vi "NumberOfPhases.vi"(11 "Device(s)Settings":T1 {"Phase Select" items=["Phase ALL", "Phase A", "Phase B", "Phase C"]}) -> (2 "Numeric Indicator":i32, 3 "Error Out":errorcluster, 5 "Boolean":bool)   [LabVIEW 2018, in "AcPwrPlugins.lvlib" / "NHRDCPower.lvclass"]
uses:
  NHRDCPower.lvclass
  TypeDefs/Device(s)Settings.ctl
  <vilib>/Utility/error.llb/Error Cluster From Error Code.vi
  <vilib>/ErrorRing/Error Ring.xnode
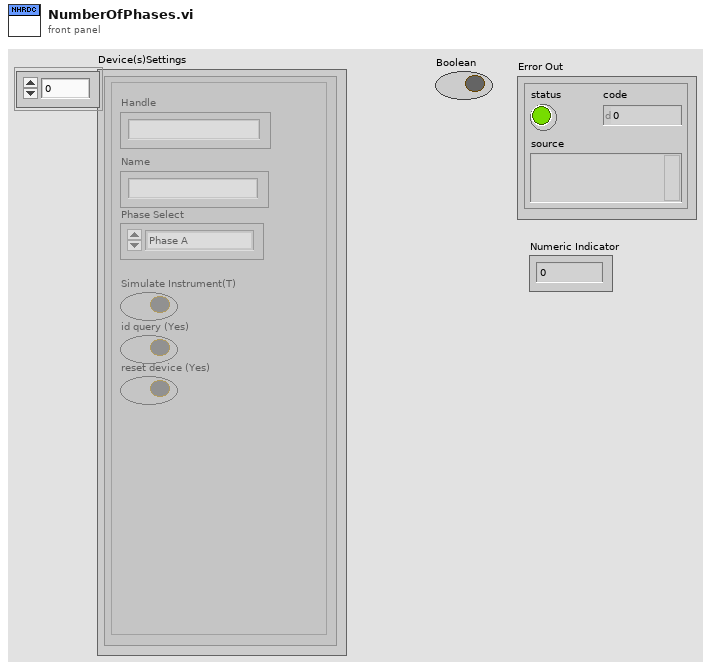
[diagram p1: front panel]
types:
  T1 = typedef "AcPwrPlugins.lvlib/NHRDCPower.lvclass/Device(s)Settings.ctl" = cluster{"Handle":string, "Name":string, "Phase Select":i32, "id query (Yes)":bool, "reset device (Yes)":bool, "Connected":bool, "Voltage Range (V)":dbl[], "Timing":cluster{"TimingOn":enum16{""}, "Hours":u32, "Minutes":u32, "Seconds":dbl, "CutoffVoltage":dbl}, "Simulate Instrument(T)":bool}[]
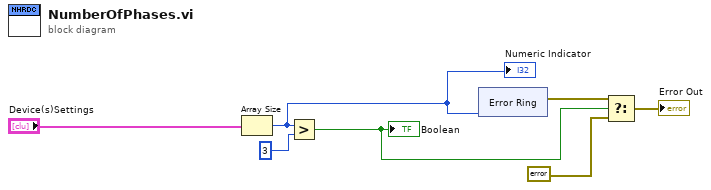
[diagram p0: block diagram]
diagram:
  n1 = Array Size(array="Device(s)Settings") -> (size(s)=w7:i32)
  "Numeric Indicator" <- w7
  n2 = Greater?(x=w7, y=3) -> (0:w3:bool)
  "Boolean" <- w3
  n3 = xnode "Error Ring"("parameter 0"=w7) -> ("error out"=w6:errorcluster)
  n4 = Select(t=w6, s=w3, f=errorcluster {"status"=FALSE, "code"=0, "source"=""}) -> (s? t:f=→"Error Out":errorcluster)
